vi "ZoomscanVI.vi"() -> ()   [LabVIEW 2025]
uses:
  <vilib>/Analysis/1siggen.llb/Ramp Pattern by Samples.vi
  <vilib>/DAQmx/write.llb/DAQmx Write (Analog 1D Wfm NChan NSamp).vi
  <vilib>/DAQmx/read.llb/DAQmx Read (Counter 1D U32 1Chan NSamp).vi
  <vilib>/DAQmx/create/channels.llb/DAQmx Create Channel (AO-Voltage-Basic).vi
  <vilib>/DAQmx/configure/timing.llb/DAQmx Timing (Sample Clock).vi
  <vilib>/DAQmx/miscellaneous.llb/DAQmx Fill In Error Info.vi
  <vilib>/DAQmx/create/channels.llb/DAQmx Create Channel (CI-Count Edges).vi
  <vilib>/Analysis/NI_AALBase.lvlib
panel:
  in  "file (use dialog)":path=path "C:/Users/admin/Documents/PVJ/Msc/Confocal and NV centers/data for scans/scan3.raw"
  out "Min Vy":dbl
  out "Max Vy":dbl
  out "Min Vx":dbl
  out "Max Vx":dbl
  out "Intensity Graph":dbl[][](graph)
  out "appended array":dbl[][](array[numeric])
  out "transposed array":dbl[][](array[numeric])
  out "64bit integer":i64[](array[numeric])
  in  "Dwell time (s)":dbl
  in  "new px":i32=128
  in  "Around desired spot":i32=128
  in  "Y coordinate":i32
  in  "X coordinate":i32
  in  "old px":i32=128
  in  "Volts":dbl=10.0 format="%0.2f"
  # "80 nm ppx"
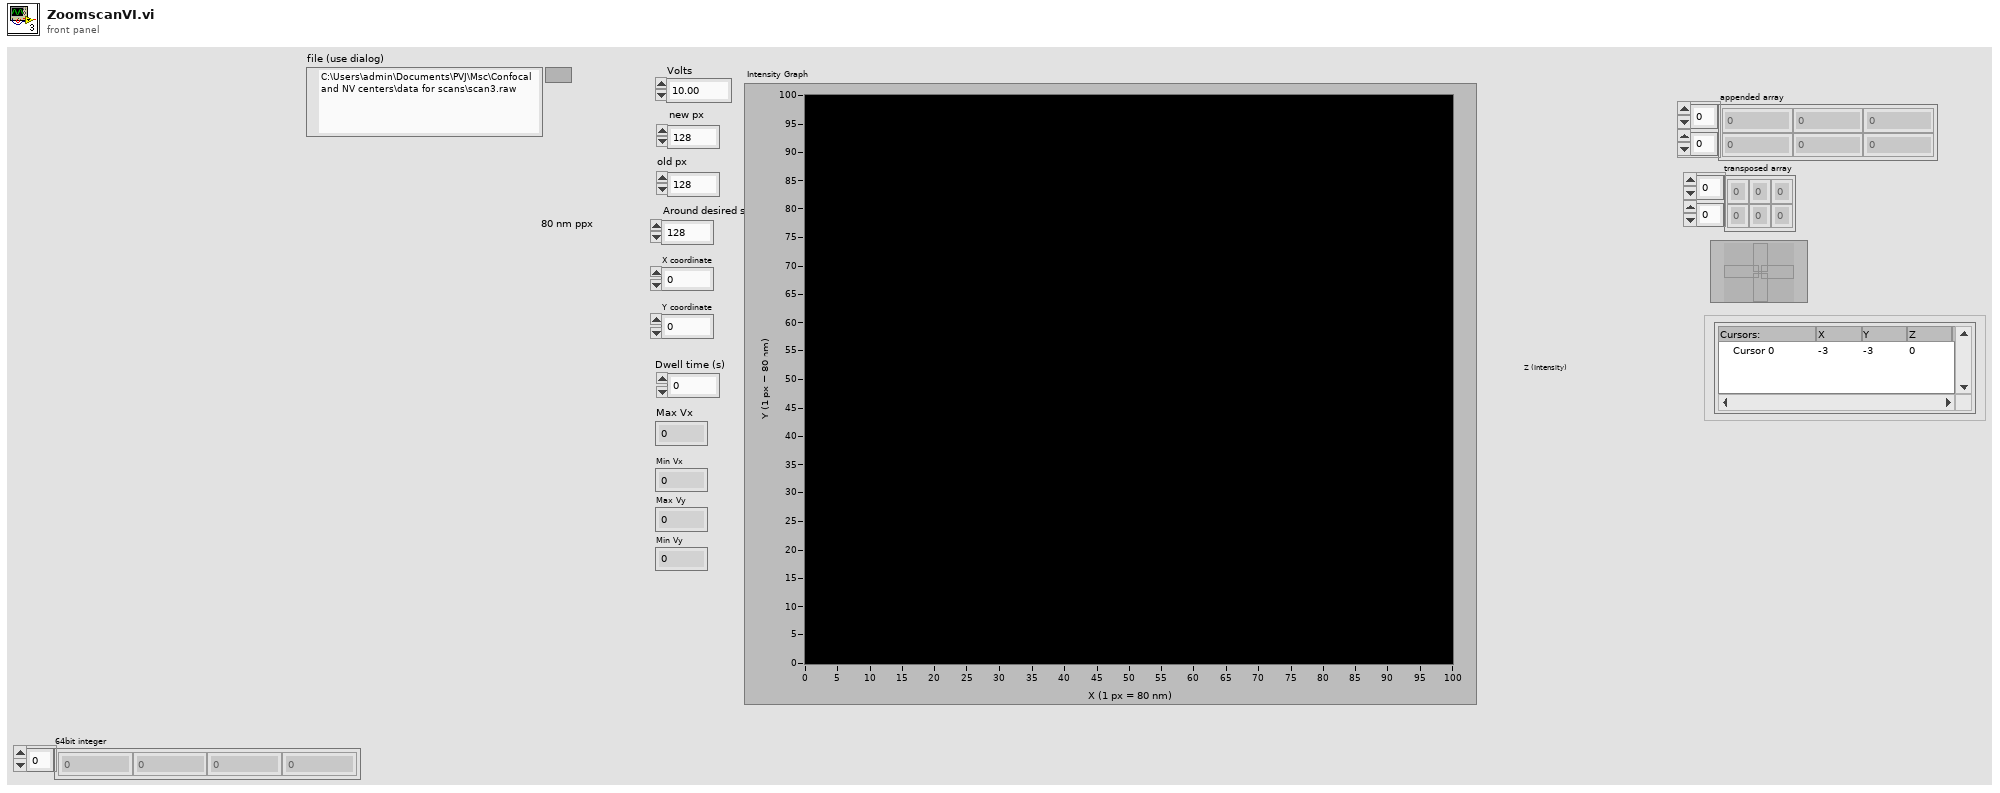
[diagram p1: front panel]
types:
  T1 = enum16{"big-endian, network order", "native, host order", "little-endian"}
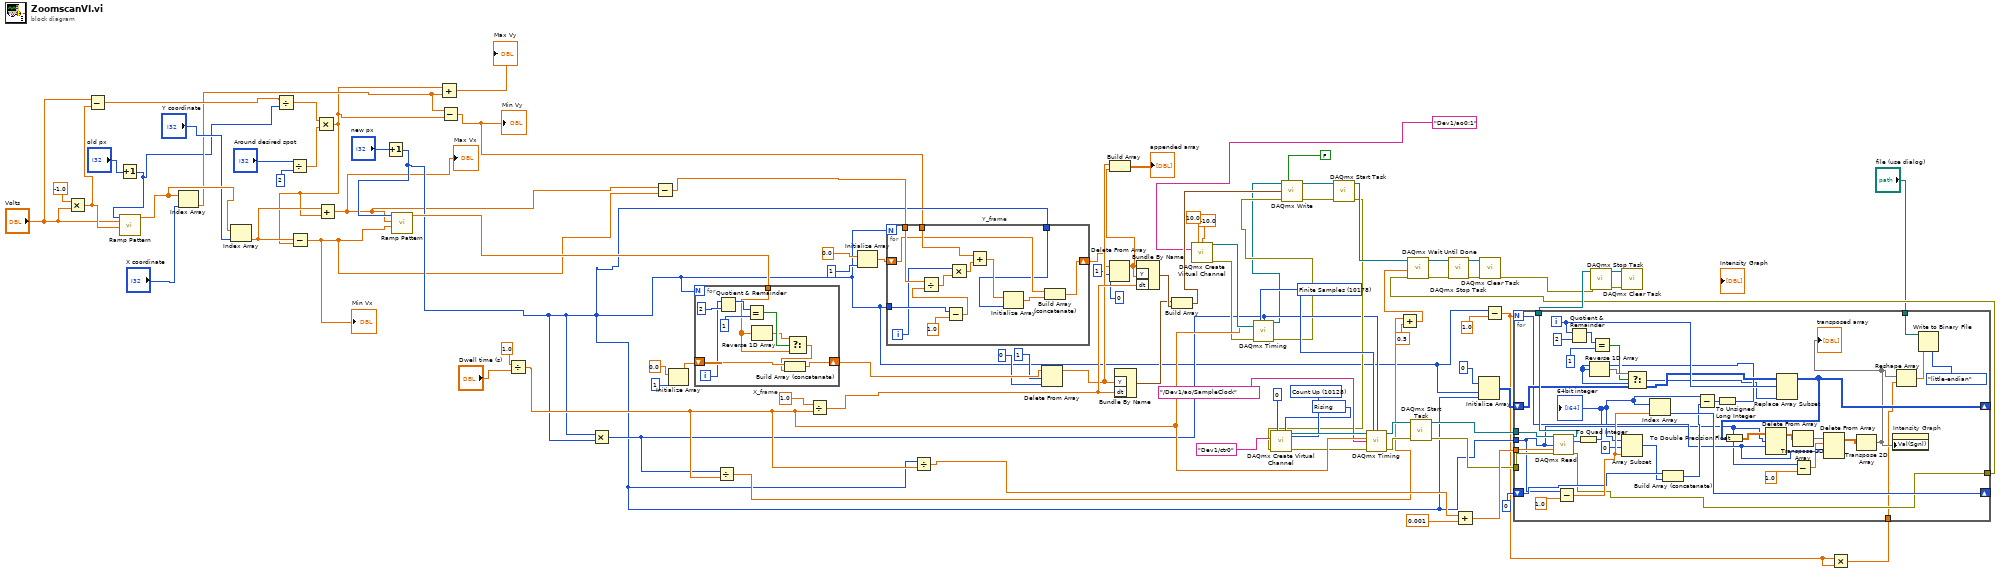
[diagram p0: block diagram]
diagram:
  w76 = 10178 items=["Finite Samples"=10178, "Continuous Samples"=10123, "Hardware Timed Single Point"=12522] ("Sample mode")
  w56 = 10280 items=["Rising"=10280, "Falling"=10171] ("edge")
  w57 = 10128 items=["Count Up"=10128, "Count Down"=10124, "Externally Controlled"=10326] ("count direction")
  n1 = Multiply(x=-1.0, y="Volts") -> (x*y=w88:dbl)
  n2 = Subtract(x="Volts", y=w88) -> (x-y=w86:dbl)
  n3 = Increment(x="old px") -> (x+1=w5:i32)
  n4 = call-poly <vilib>:"Ramp Pattern.vi"("start"=w88, "end"="Volts", "samples"=w5) -> ("Ramp Pattern"=w92:dbl[])  [unwired: 7 in, 1 out]
  n5 = Index Array(array=w92, index="X coordinate") -> (element=w14:dbl)
  n6 = Index Array(array=w92, index="Y coordinate") -> (element=w16:dbl)
  n7 = Divide(x=w86, y=w5) -> (x/y=w85:dbl)
  n8 = Divide(x="Around desired spot", y=2) -> (x/y=w84:dbl)
  n9 = Multiply(x=w85, y=w84) -> (x*y=w13:dbl)
  n10 = Subtract(x=w16, y=w13) -> (x-y=w9:dbl)
  "Min Vx" <- w9
  n11 = Add(x=w16, y=w13) -> (x+y=w15:dbl)
  "Max Vx" <- w15
  n12 = Increment(x="new px") -> (x+1=w17:i32)
  n13 = call-poly <vilib>:"Ramp Pattern.vi"("start"=w9, "end"=w15, "samples"=w17) -> ("Ramp Pattern"=w18:dbl[])  [unwired: 7 in, 1 out]
  n14 = Add(x=w13, y=w14) -> (x+y=→"Max Vy":dbl)
  n15 = Subtract(x=w14, y=w13) -> (x-y=w8:dbl)
  "Min Vy" <- w8
  n16 = Divide(x=1.0, y="Dwell time (s)") -> (x/y=w41:dbl)
  n17 = Multiply(x=w17, y=w17) -> (x*y=w25:i32)
  n18 = Subtract(x=w15, y=w9) -> (x-y=w20:dbl)
  n19 = Initialize Array(0.0 ("element"), 1 ("dimension size")) -> (w64:dbl[])
  n20 = for "X_frame" {
    N: w17 -> [_]
    shift-right: [w103] -> w52
    shift-left: w64 -> [w104]
    tunnel: w18 -> [w97]
    i -> [w98]
    n21 = Quotient & Remainder(x=w98, y=2) -> (x-y*floor(x/y)=w101:i32)  [unwired: 1 out]
    n22 = Equal?(x=w101, y=1) -> (x = y?=w99:bool)
    n23 = Reverse 1D Array(array=w97) -> (reversed array=w96:dbl[])
    n24 = Select(t=w96, s=w99, f=w97) -> (s? t:f=w95:dbl[])
    n25 = Build Array (concatenate)(w104, w95) -> (w103:dbl[])
  }
  n26 = Divide(x=w25, y=w41) -> (x/y=w24:dbl)
  n27 = Divide(x=1.0, y=w41) -> (x/y=w66:dbl)
  n28 = Initialize Array(0.0 ("element"), 1 ("dimension size")) -> (w65:dbl[])
  n29 = for "Y_frame" {
    N: w17 -> [_]
    tunnel: w17 -> [w117]
    tunnel: w20 -> [w115]
    tunnel: w8 -> [w110]
    tunnel: w17 -> [w105]
    shift-right: [w106] -> w48
    shift-left: w65 -> [w107]
    i -> [w112]
    n30 = Subtract(x=w117, y=1.0) -> (x-y=w114:dbl)
    n31 = Divide(x=w115, y=w114) -> (x/y=w113:dbl)
    n32 = Multiply(x=w112, y=w113) -> (x*y=w111:dbl)
    n33 = Add(x=w110, y=w111) -> (x+y=w109:dbl)
    n34 = Initialize Array(w109, w105) -> (w108:dbl[])
    n35 = Build Array (concatenate)(w107, w108) -> (w106:dbl[])
  }
  n36 = Divide(x=w17, y=w41) -> (x/y=w38:dbl)
  n37 = Delete From Array "Delete From Array"(array=w52, length=1, index=0) -> (array with subset deleted=w49:dbl[])  [unwired: 1 out]
  n38 = Delete From Array "Delete From Array"(array=w48, length=1, index=0) -> (array with subset deleted=w42:dbl[])  [unwired: 1 out]
  n39 = Build Array(w49, w42) -> (→"appended array":dbl[][])
  n40 = Bundle By Name("Y"=w49, "dt"=w66) -> (w67:waveform(dbl))  [unwired: 1 in]
  n41 = Bundle By Name("Y"=w42, "dt"=w66) -> (w68:waveform(dbl))  [unwired: 1 in]
  n42 = Build Array(w67, w68) -> (w70:waveform(dbl)[])
  n43 = call-poly <vilib>:"DAQmx Create Virtual Channel.vi"("maximum value"=10.0, "minimum value"=-10.0, "physical channels"="Dev1/ao0:1" ("Galvo mirror path")) -> ("task out"=w69:refnum<k21>, "error out"=w36:errorcluster)  [unwired: 11 in]
  n44 = call-poly <vilib>:"DAQmx Timing.vi"("task/channels in"=w69, "sample mode"=w76, "samples per channel"=w25, "rate"=w41, "error in"=w36) -> ("task out"=w6:refnum<k21>, "error out"=w7:errorcluster)  [unwired: 9 in]
  n45 = call-poly <vilib>:"DAQmx Write.vi"("task/channels in"=w6, "auto start"=FALSE, "data"=w70, "error in"=w7) -> ("task out"=w71:refnum<k21>, "error out"=w35:errorcluster)  [unwired: 9 in, 1 out]
  n46 = call <vilib>:"DAQmx Start Task.vi"("task/channels in"=w71, "error in"=w35) -> ("task out"=w78:refnum<k21>, "error out"=w32:errorcluster)  [unwired: 12 in]
  n47 = call-poly <vilib>:"DAQmx Create Virtual Channel.vi"("initial count"=u32 0, "count direction"=w57, "edge"=w56, "counter"="Dev1/ctr0" ("Counter path"), "error in"=w32) -> ("task out"=w73:refnum<k21>, "error out"=w34:errorcluster)  [unwired: 9 in]
  n48 = call-poly <vilib>:"DAQmx Timing.vi"("task/channels in"=w73, "sample mode"=w76, "samples per channel"=w25, "rate"=w41, "source"=tag "/Dev1/ao/SampleClock", "error in"=w34) -> ("task out"=w74:refnum<k21>, "error out"=w33:errorcluster)  [unwired: 8 in]
  n49 = Add(x=w24, y=0.5) -> (x+y=w22:dbl)
  n50 = call <vilib>:"DAQmx Start Task.vi"("task/channels in"=w74, "error in"=w33) -> ("task out"=w75:refnum<k21>, "error out"=w27:errorcluster)  [unwired: 12 in]
  n51 = Add(x=w38, y=0.001) -> (x+y=w43:dbl)
  n52 = Initialize Array(u32 0 ("element"), w17, w17) -> (w77:u32[][])
  n53 = Subtract(x=w17, y=1.0) -> (x-y=w2:dbl)
  n54 = Multiply(x=w2, y=w2) -> (x*y=w1:dbl)
  n55 = for {
    N: w2 -> [w128]
    tunnel: w17 -> [w125]
    tunnel: w43 -> [w155]
    tunnel: w75 -> [w154]
    shift-right: [w137] -> _
    shift-left: w77 -> [w140]
    tunnel: [w149] -> w37
    shift-right: [w146] -> _
    shift-left: u64 0 ("Numeric") -> [w144]
    tunnel: w27 -> [w135]
    tunnel: [w134] -> w26
    tunnel: "file (use dialog)" -> [w121]
    tunnel: w1 -> [w118]
    i -> [w141]
    n56 = call-poly <vilib>:"DAQmx Read.vi"("task/channels in"=w154, "number of samples per channel"=w125, "timeout"=w155, "error in"=w135) -> ("task out"=w149:refnum<k21>, "data"=w136:u32[], "error out"=w134:errorcluster)  [unwired: 9 in]
    n57 = Subtract(x=w125, y=1.0) -> (x-y=w145:dbl)
    n58 = Quotient & Remainder(x=w141, y=2) -> (x-y*floor(x/y)=w152:i32)  [unwired: 1 out]
    n59 = To Quad Integer(1:w136) -> (0:w123:i64[])
    "64bit integer" <- w123
    n60 = Equal?(x=w152, y=1) -> (x = y?=w148:bool)
    n61 = Array Subset "Array Subset"(array=w123, index=0, length=w145) -> (w124:i64[])
    n62 = Index Array "Index Array"(array=w123, index=w145) -> (element=w146:i64)
    n63 = Build Array (concatenate) "Build Array"(w144, w124) -> (w143:u64[])
    n64 = Subtract(x=w123, y=w143) -> (x-y=w142:u64[])
    n65 = To Unsigned Long Integer(number=w142) -> (unsigned 32bit integer=w139:u32[])
    n66 = Reverse 1D Array(array=w139) -> (reversed array=w150:u32[])
    n67 = Select(t=w150, s=w148, f=w139) -> (s? t:f=w138:u32[])
    n68 = Replace Array Subset "Replace Array Subset"(array=w140, new element=w138, index (row)=w141) -> (w137:u32[][])  [unwired: 1 in]
    n69 = To Double Precision Float(number=w137) -> (double precision float=w133:dbl[][])
    n70 = Delete From Array(array=w133, length=w125, index (row)=w128) -> (array with subset deleted=w132:dbl[][])  [unwired: 1 in, 1 out]
    n71 = Transpose 2D Array(2D array=w132) -> (transposed array=w131:dbl[][])
    n72 = Subtract(x=w125, y=1.0) -> (x-y=w129:dbl)
    n73 = Delete From Array(array=w131, length=w129, index (row)=w128) -> (array with subset deleted=w127:dbl[][])  [unwired: 1 in, 1 out]
    n74 = Transpose 2D Array(2D array=w127) -> (transposed array=w122:dbl[][])
    "transposed array" <- w122
    n75 = property on="Intensity Graph" class="IntGraph (strict)"("Val(Sgnl)"=w122) -> ()  [unwired: 2 in, 2 out]
    n76 = Reshape Array(w122, w118) -> (w119:dbl[])
    n77 = Write to Binary File(file (use dialog)=w121, data=w119, 9:T1."little-endian" ("byte order (0:big-endian, network order)")) -> ()  [unwired: 3 in, 3 out]
  }
  n78 = call <vilib>:"DAQmx Wait Until Done.vi"("task/channels in"=w78, "timeout (sec)"=w22, "error in"=w26) -> ("task out"=w79:refnum<k21>, "error out"=w31:errorcluster)  [unwired: 11 in]
  n79 = call <vilib>:"DAQmx Stop Task.vi"("task/channels in"=w79, "error in"=w31) -> ("task out"=w72:refnum<k21>, "error out"=w30:errorcluster)  [unwired: 12 in]
  n80 = call <vilib>:"DAQmx Clear Task.vi"("task in"=w72, "error in"=w30) -> ("error out"=w29:errorcluster)  [unwired: 13 in]
  n81 = call <vilib>:"DAQmx Stop Task.vi"("task/channels in"=w37, "error in"=w29) -> ("task out"=w80:refnum<k21>, "error out"=w28:errorcluster)  [unwired: 12 in]
  n82 = call <vilib>:"DAQmx Clear Task.vi"("task in"=w80, "error in"=w28) -> ()  [unwired: 13 in, 1 out]
